vi "noise.vi"() -> ()   [LabVIEW 2009]
uses:
  <vilib>/Analysis/NI_AALBase.lvlib
panel:
  out "歪み率":dbl
  out "XYグラフ":cluster{dbl[], dbl[]}(graph)
  in  "位相":dbl
  in  "Q":dbl
  out "送信波":cluster{dbl[], dbl[]}(graph)
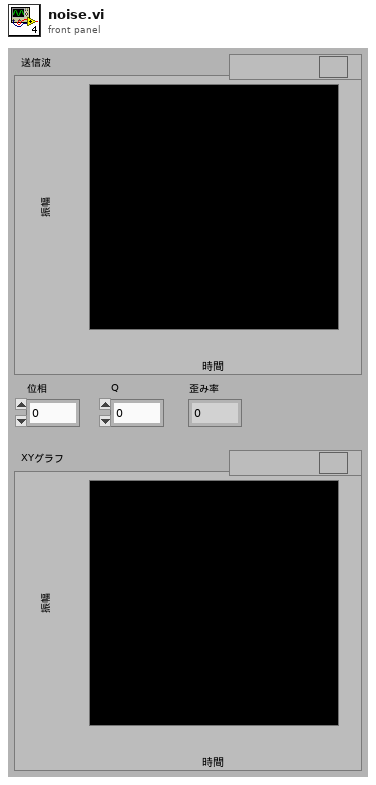
[diagram p1: front panel]
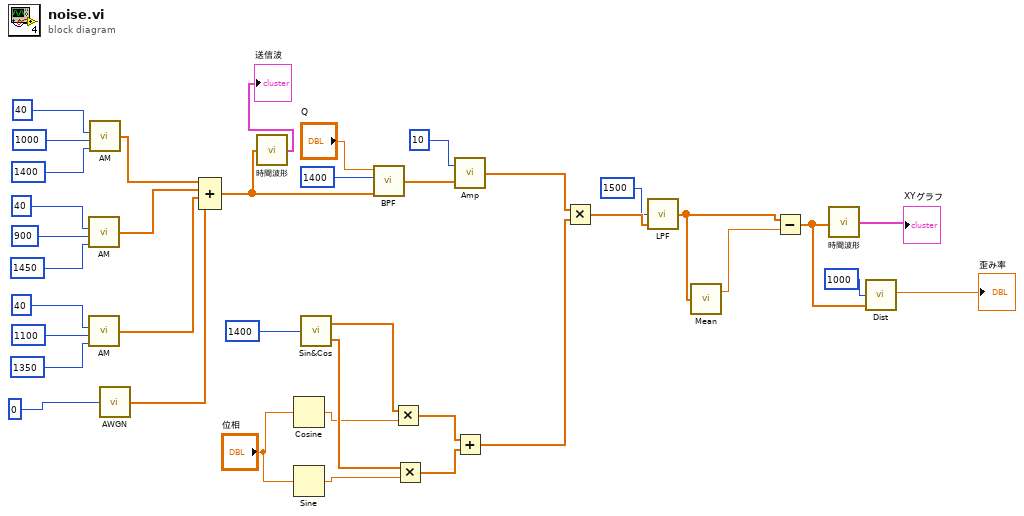
[diagram p0: block diagram]
diagram:
  n1 = call "AM.vi"("変調度 [%]"=40, "変調周波数 [Hz]"=900, "搬送波周波数 [kHz]"=1450) -> ("変調波"=w28:dbl[])  [unwired: 2 in]
  n2 = call "AM.vi"("変調度 [%]"=40, "変調周波数 [Hz]"=1100, "搬送波周波数 [kHz]"=1350) -> ("変調波"=w27:dbl[])  [unwired: 2 in]
  n3 = call "AM.vi"("変調度 [%]"=40, "変調周波数 [Hz]"=1000, "搬送波周波数 [kHz]"=1400) -> ("変調波"=w29:dbl[])  [unwired: 2 in]
  n4 = call "AWGN.vi"("振幅値"=0) -> ("出力"=w26:dbl[])
  n5 = Compound Arithmetic op=ADD(w29, w28, w27, w26) -> (w23:dbl[])
  n6 = call "時間波形.vi"("入力"=w23) -> ("時間波形"=→"送信波":cluster{dbl[], dbl[]})
  n7 = Cosine(x="位相") -> (cos(x)=w3:dbl)
  n8 = Sine(x="位相") -> (sin(x)=w1:dbl)
  n9 = call "Sin&Cos.vi"("周波数[kHz]"=1400) -> ("sin"=w13:dbl[], "cos"=w12:dbl[])
  n10 = call "BPF.vi"("X"=w23, "中心周波数 [kHz]"=1400, "Q"="Q") -> ("BPF出力"=w21:dbl[])  [unwired: 1 in]
  n11 = Multiply(x=w13, y=w3) -> (x*y=w11:dbl[])
  n12 = Multiply(x=w12, y=w1) -> (x*y=w10:dbl[])
  n13 = call "Amp.vi"("入力"=w21, "増幅率"=10) -> ("出力"=w18:dbl[])
  n14 = Add(x=w11, y=w10) -> (x+y=w9:dbl[])
  n15 = Multiply(x=w18, y=w9) -> (x*y=w17:dbl[])
  n16 = call "LPF.vi"("入力"=w17, "カットオフ周波数 [Hz]"=1500) -> ("LPF出力"=w7:dbl[])  [unwired: 1 in]
  n17 = call <vilib>:"Mean.vi"("X"=w7) -> ("mean"=w8:dbl)  [unwired: 1 out]
  n18 = Subtract(x=w7, y=w8) -> (x-y=w6:dbl[])
  n19 = call "時間波形.vi"("入力"=w6) -> ("時間波形"=→"XYグラフ":cluster{dbl[], dbl[]})
  n20 = call "Dist.vi"("入力"=w6, "基本周波数 [Hz]"=1000) -> ("ひずみ率"=→"歪み率":dbl)  [unwired: 1 in]
